vi "WS1050 OFFSET CAL.vi"(8 "error in":errorcluster, 10 "OFFSET CAL":bool=TRUE) -> (0 "error out":errorcluster, 3 "AD7747 Values":string[][](table))   [LabVIEW 2012]
uses:
  Type Defs/WSVCAP SHL I2C DUT Mask Mode Enum.ctl
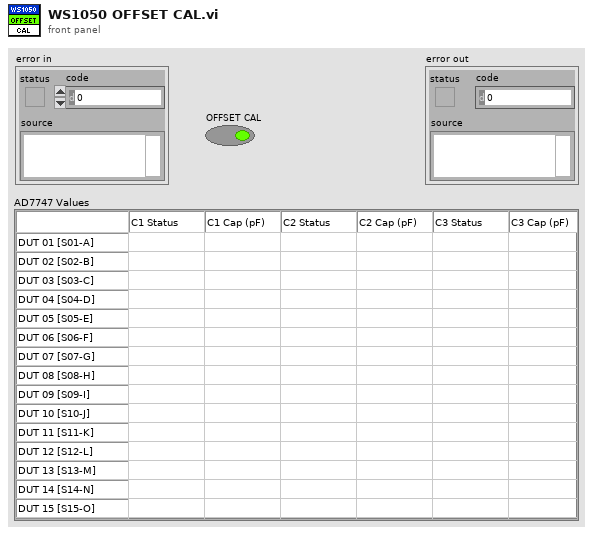
[diagram p1: front panel]
types:
  T1 = typedef "WSVCAP SHL I2C DUT Mask Mode Enum.ctl" = enum16{"Custom", "C1", "C2", "C3", "All"}
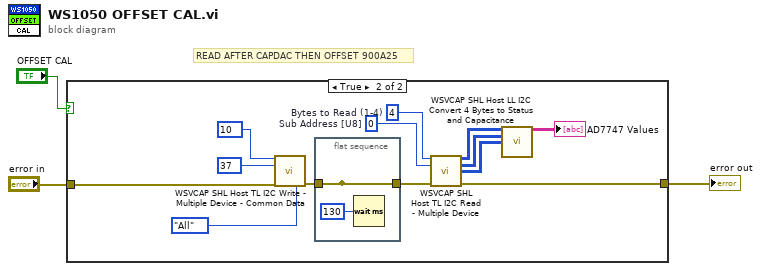
[diagram p0: block diagram]
diagram:
  # "READ AFTER CAPDAC THEN OFFSET 900A25"
  n1 = case shown="True" "OFFSET CAL" {
    tunnel: "error in" -> [w4 w17]
    tunnel: [w4 w8] -> w3
    frame False {
    }
    frame True {
      w14 = u8 4  # Bytes to Read (1-4)
      w15 = u8 0  # Sub Address [U8]
      n2 = call "WSVCAP SHL Host TL I2C Write - Multiple Device - Common Data.vi"("Sub Address"=u8 10, "Data Out [U8]"=u8 37 ("Sub Address"), "error in"=w17, "DUT Mask Mode (All)"=WSVCAP_SHL_I2C_DUT_Mask_Mode_Enum."All") -> ("error out"=w16:errorcluster)  [unwired: 11 in]
      n3 = flat-sequence {
        tunnel: w16 -> [w18]
        tunnel: [w18] -> _
        tunnel: [w18] -> w9
        frame #0 {
          n4 = Wait (ms)(milliseconds to wait=u32 130) -> ()  [unwired: 1 out]
        }
      }
      n5 = call "WSVCAP SHL Host TL I2C Read - Multiple Device.vi"("Bytes to Read (1-4)"=w14, "Sub Address [U8]"=w15, "error in"=w9) -> ("C1:1-16 Read Data [U8]"=w13:u8[][], "C2:1-16 Read Data [U8]"=w12:u8[][], "C3:1-16 Read Data [U8]"=w10:u8[][], "error out"=w8:errorcluster)  [unwired: 9 in]
      n6 = call "WSVCAP SHL Host LL I2C Convert 4 Bytes to Status and Capacitance.vi"("C1:1-16 Read Data [U8]"=w13, "C2_1-16 Read Data [U8]"=w12, "C3_1-16 Read Data [U8]"=w10) -> ("AD7747 Values"=→"AD7747 Values":string[][])  [unwired: 12 in]
    }
  }
  "error out" <- w3
